vi "test_MonoMoveToPosition.vi"(0 "device selection":enum16{"monochromator", "CCD", "SCD"}(ring)=enum."CCD", 1 "Test should pass":bool=TRUE, 5 "set-up a connection":bool=TRUE, 9 "tear down connection":bool=TRUE, 11 "error in":errorcluster, 12 "Delay between send and receive [ms]":i32=100, 13 "wait for procedure to be finished [ms]":i32=15000) -> (10 "log-file path":path, 15 "error out":errorcluster)   [LabVIEW 2023]
uses:
  Classes/Mono/Monochromator.lvclass
  <vilib>/addons/_JKI Toolkits/Caraya/classes/Assert/Assert Equal Value and Type_Variant.vi
  <vilib>/addons/_JKI Toolkits/Caraya/classes/Assert/Assert Not Error.vi
  <vilib>/addons/_JKI Toolkits/Caraya/classes/Test/Test.lvclass
  <vilib>/addons/_JKI Toolkits/Caraya/classes/Assert/Assert.lvclass
panel:
  # "Connector Pane"
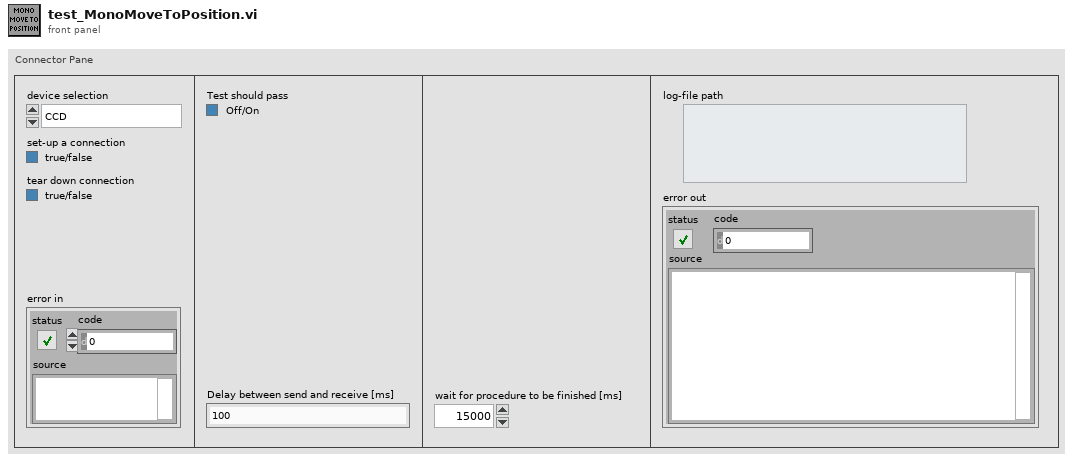
[diagram p1: front panel]
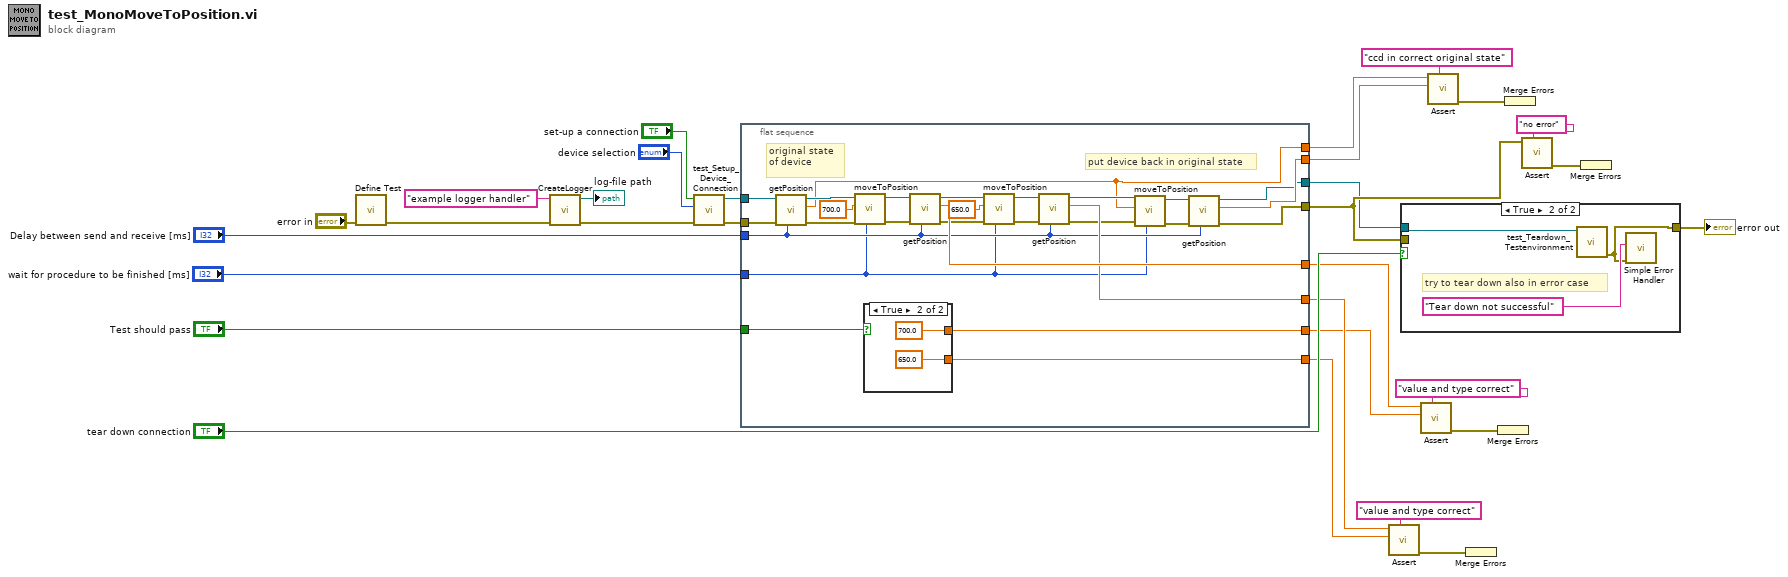
[diagram p0: block diagram]
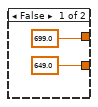
[diagram p2: hidden frame]
diagram:
  n1 = call <vilib>:"Define Test.vi"("error in (no error)"="error in") -> ("error out"=w2:errorcluster)  [unwired: 9 in, 1 out]
  n2 = call "CreateLogger.vi"("error in (no error)"=w2, "Handler Name"="example logger handler") -> ("error out"=w1:errorcluster, "log-file path"=→"log-file path":path)  [unwired: 8 in]
  n3 = call "test_Setup_Device_Connection.vi"("error in (no error)"=w1, "device selection"="device selection", "set-up a connection"="set-up a connection") -> ("error out"=w8:errorcluster, "Monochromator.lvclass"=w6:refnum<class "Monochromator.lvclass">)  [unwired: 5 in, 2 out]
  n4 = flat-sequence {
    tunnel: w8 -> [w53]
    tunnel: w6 -> [w54]
    tunnel: [w33] -> w21
    tunnel: "Test should pass" -> [w57]
    tunnel: [w34] -> w20
    tunnel: [w41] -> w19
    tunnel: [w56] -> w18
    tunnel: [w47] -> w17
    tunnel: [w55] -> w16
    tunnel: [w36] -> w13
    tunnel: [w35] -> w12
    tunnel: "Delay between send and receive [ms]" -> [w32]
    tunnel: "wait for procedure to be finished [ms]" -> [w31]
    frame #0 {
      # "put device back in original state"
      # "original state of device"
      n5 = call "getPosition.vi"("Delay between send and receive [ms]"=w32, "error in (no error)"=w53, "Monochromator in"=w54) -> ("error out"=w51:errorcluster, "wavelength"=w36:dbl, "Monochromator out"=w52:refnum<class "Monochromator.lvclass">)  [unwired: 6 in]
      n6 = call "moveToPosition.vi"("Delay between send and receive [ms]"=w31, "error in (no error)"=w51, "wavelength"=700.0 ("exposure time [ms]"), "Monochromator in"=w52) -> ("error out"=w49:errorcluster, "Monochromator out"=w48:refnum<class "Monochromator.lvclass">)  [unwired: 4 in, 2 out]
      n7 = case shown="True" w57 {
        tunnel: [649.0 ("exposure time [ms]") 650.0 ("exposure time [ms]")] -> w56
        tunnel: [699.0 ("exposure time [ms]") 700.0 ("exposure time [ms]")] -> w55
        frame False {
        }
        frame True {
        }
      }
      n8 = call "getPosition.vi"("Delay between send and receive [ms]"=w32, "error in (no error)"=w49, "Monochromator in"=w48) -> ("error out"=w43:errorcluster, "wavelength"=w47:dbl, "Monochromator out"=w44:refnum<class "Monochromator.lvclass">)  [unwired: 6 in]
      n9 = call "moveToPosition.vi"("Delay between send and receive [ms]"=w31, "error in (no error)"=w43, "wavelength"=650.0 ("exposure time [ms]"), "Monochromator in"=w44) -> ("error out"=w46:errorcluster, "Monochromator out"=w45:refnum<class "Monochromator.lvclass">)  [unwired: 4 in, 2 out]
      n10 = call "getPosition.vi"("Delay between send and receive [ms]"=w32, "error in (no error)"=w46, "Monochromator in"=w45) -> ("error out"=w38:errorcluster, "wavelength"=w41:dbl, "Monochromator out"=w39:refnum<class "Monochromator.lvclass">)  [unwired: 6 in]
      n11 = call "moveToPosition.vi"("Delay between send and receive [ms]"=w31, "error in (no error)"=w38, "wavelength"=w36, "Monochromator in"=w39) -> ("error out"=w40:errorcluster, "Monochromator out"=w37:refnum<class "Monochromator.lvclass">)  [unwired: 4 in, 2 out]
      n12 = call "getPosition.vi"("Delay between send and receive [ms]"=w32, "error in (no error)"=w40, "Monochromator in"=w37) -> ("error out"=w33:errorcluster, "wavelength"=w35:dbl, "Monochromator out"=w34:refnum<class "Monochromator.lvclass">)  [unwired: 6 in]
    }
  }
  n13 = call-poly <vilib>:"Assert.vi"("Label"="value and type correct" ("Label (VI Title)"), "Y"=w18, "X"=w19) -> ("error out"=w29:errorcluster)  [unwired: 7 in, 1 out]
  n14 = case shown="True" "tear down connection" {
    tunnel: w20 -> [_ w64]
    tunnel: [w62 w63] -> w11
    tunnel: w21 -> [w62 _]
    frame False {
    }
    frame True {
      # "try to tear down also in error case"
      n15 = call "test_Teardown_Testenvironment.vi"("GenericDevice.lvclass"=w64) -> ("error out"=w63:errorcluster)  [unwired: 9 in, 1 out]
      n16 = call <vilib>:"Simple Error Handler.vi"("error source (\" \")"="Tear down not successful" ("error source (\" \")"), "error in (no error)"=w63) -> ()  [unwired: 3 in, 5 out]
    }
  }
  "error out" <- w11
  n17 = call-poly <vilib>:"Assert.vi"("Label"="value and type correct" ("Label (VI Title)"), "Y"=w16, "X"=w17) -> ("error out"=w28:errorcluster)  [unwired: 7 in, 1 out]
  n18 = call-poly <vilib>:"Assert.vi"("Label"="ccd in correct original state" ("Label (VI Title)"), "Y"=w12, "X"=w13) -> ("error out"=w15:errorcluster)  [unwired: 7 in, 1 out]
  n19 = Merge Errors(w29) -> ()  [unwired: 1 out]
  n20 = Merge Errors(w28) -> ()  [unwired: 1 out]
  n21 = Merge Errors(w15) -> ()  [unwired: 1 out]
  n22 = call-poly <vilib>:"Assert.vi"("Label"="no error" ("Label (VI Title)"), "Not Error?"=w21) -> ("error out"=w23:errorcluster)  [unwired: 8 in, 1 out]
  n23 = Merge Errors(w23) -> ()  [unwired: 1 out]
